vi "LVClass_DataServer SetString.vi"(0 "DataServer in":refnum<class "DataServer.lvclass">, 5 "name":string, 7 "Value":string, 11 "error in (no error)":errorcluster) -> (4 "DataServer out":refnum<class "DataServer.lvclass">, 15 "error out":errorcluster)   [LabVIEW 2020, in "DataServer.lvclass"]
doc: "Set data corresponding to /p name.\n\n<B>serverIn</B> : Server object.\n<B>serverOut</B> : Server object.\n<B>name</B> : Data name\n<B>data</B> : Data value"
uses:
  DataServer.lvclass
  DataServer.lvclass/DataServer.ctl
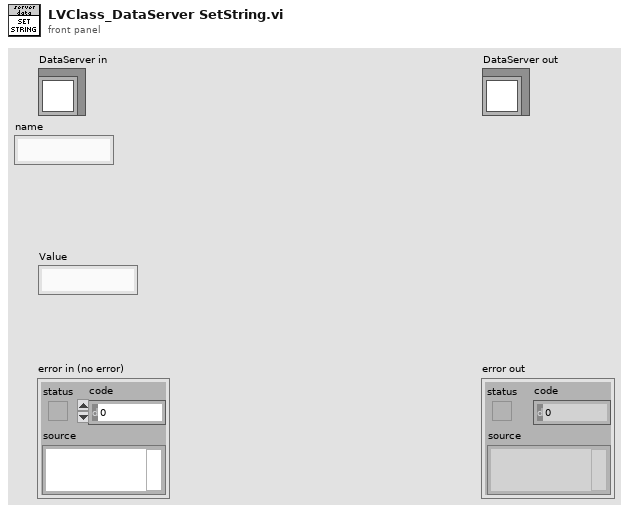
[diagram p1: front panel]
types:
  T1 = typedef "ClassID.ctl" = i64
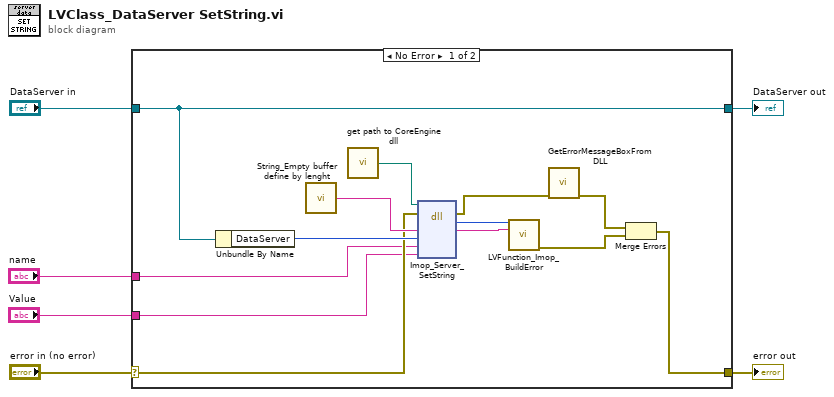
[diagram p0: block diagram]
diagram:
  n1 = case shown="No Error" "error in (no error)" {
    selector: "error in (no error)" -> [w10 w21]
    tunnel: [w9 w21] -> w5
    tunnel: [w11 w20] -> w3
    tunnel: "DataServer in" -> [w11 w20]
    tunnel: "Value" -> [w7 _]
    tunnel: "name" -> [w8 _]
    frame No Error {
      n2 = Unbundle By Name(w11) -> ("DataServer"=w17:T1)
      n3 = call "String_Empty buffer define by lenght.vi"() -> ("Empty buffer"=w14:string)  [unwired: 1 in]
      n4 = call "get path to CoreEngine dll.vi"() -> ("path to wavekit library"=w15:path)  [unwired: 14 in, 1 out]
      n5 = dll-call lib="D:/soft/HASO_v3/SVN_trunk/ImOpCoreEngine4_LV2011/DLLs/c_interface_vc100.dll" fn="Imop_Server_SetString"(path in=w15, error in=w10, "message"=w14, "server"=w17, "name"=w8, "data"=w7) -> (error out=w16:errorcluster, "return type"=w12:i32, "message"=w13:string)  [unwired: 4 in, 1 out]
      n6 = call "LVFunction_Imop_BuildError.vi"("code"=w12, "String to Prepend to source (\"\")"=w13) -> ("error out"=w19:errorcluster)  [unwired: 13 in]
      n7 = call "GetErrorMessageBoxFromDLL.vi"("error IN"=w16) -> ("error OUT"=w18:errorcluster)  [unwired: 10 in]
      n8 = Merge Errors(w18, w19) -> (w9:errorcluster)
    }
    frame Error {
    }
  }
  "error out" <- w5
  "DataServer out" <- w3
